vi "ConfigJSON_Create.vi"(0 "reference in":refnum<class "ConfigJSON.lvclass">, 5 "error in (no error)":errorcluster, 6 "Config Dir":path) -> (14 "reference out":refnum<class "ConfigJSON.lvclass">, 19 "error out":errorcluster)   [LabVIEW 2019]
doc: "Constructor."
uses:
  ConfigJSON.lvclass
  D:/LabASF/LabASF/src/ConfigInterface_class/ConfigInterface.lvclass
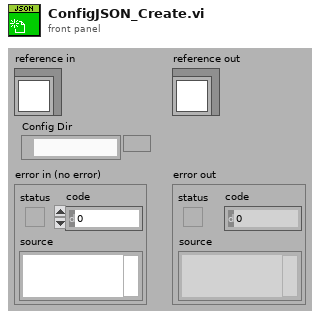
[diagram p1: front panel]
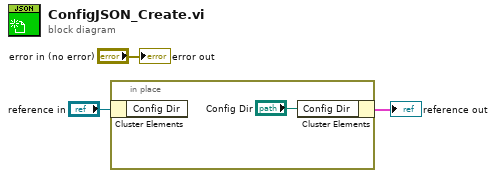
[diagram p0: block diagram]
diagram:
  n1 = in-place {
    n2 = in-place-cluster #1("reference in") -> ()  [unwired: 1 out]
    n3 = in-place-cluster #1("Config Dir"="Config Dir") -> (→"reference out":cluster{})
  }
  "error out" <- "error in (no error)"
